vi "chart title set layout.vi"(8 "error in (no error)":errorcluster, 10 "layout":T1, 11 "chart":u32) -> (0 "error out":errorcluster, 2 "layout out":T1)   [LabVIEW 8.6]
doc: "void chart_title_set_layout(lxw_chart chart, lxw_chart_layout *layout);"
uses:
  pending_lvxlsxwriter/xlsxwriter.dll
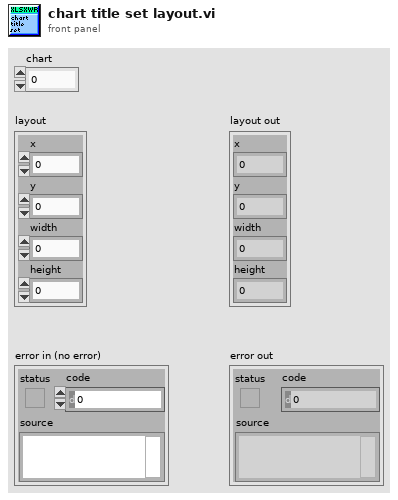
[diagram p1: front panel]
types:
  T1 = cluster{"x":dbl, "y":dbl, "width":dbl, "height":dbl}
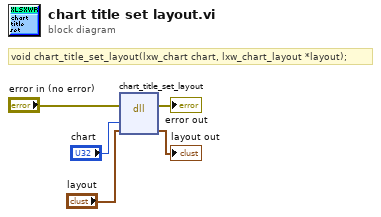
[diagram p0: block diagram]
diagram:
  # "void chart_title_set_layout(lxw_chart chart, lxw_chart_layout *layout);"
  n1 = dll-call lib="C:/Users/WDAGUtilityAccount/Desktop/pending_lvxlsxwriter/xlsxwriter.*" fn="chart_title_set_layout"(error in="error in (no error)", "chart"="chart", "layout"="layout") -> (error out=→"error out":errorcluster, "layout"=→"layout out":T1)  [unwired: 4 in, 1 out]
